vi "Set Reader Timestamp.vi"(9 "timestamp":timestamp format="%<%H:%M:%S%6u\n%x>T", 10 "ID":string="Reader", 11 "data attributes in":variant) -> (3 "data attributes out":variant)   [LabVIEW 2017]
uses:
  <vilib>/Utility/error.llb/whitespace.ctl
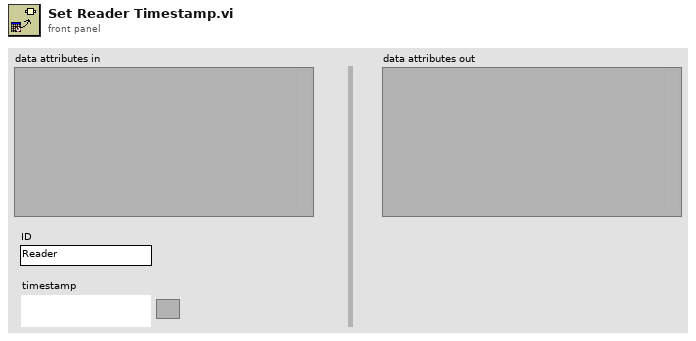
[diagram p1: front panel]
types:
  T1 = typedef "whitespace.ctl" = u16
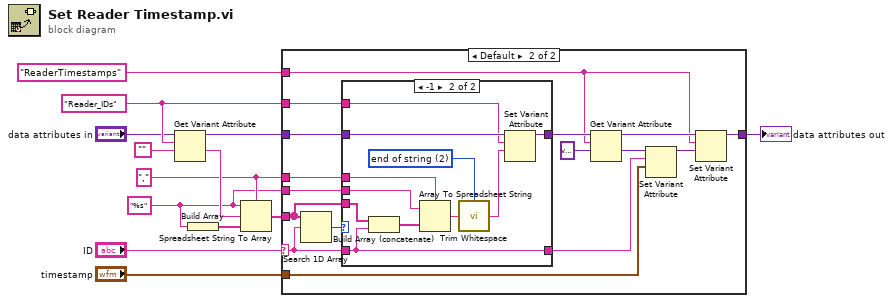
[diagram p0: block diagram]
diagram:
  w7 = "," ("delimiter (Tab)")
  w6 = "Reader_IDs" ("name")
  w5 = "%s" ("format string")
  n1 = Get Variant Attribute(Variant="data attributes in", name=w6, default value (empty Variant)="" ("name")) -> (duplicate Variant=w8:variant, value=w12:string)  [unwired: 1 in, 2 out]
  n2 = Build Array(w5) -> (w11:string[])
  n3 = Spreadsheet String To Array(delimiter (Tab)=w7, format string=w5, spreadsheet string=w12, array type (2D Dbl)=w11) -> (array=w10:string[])
  n4 = case shown="Default" "ID" {
    selector: "ID" -> [_ w27]
    tunnel: w10 -> [_ w28]
    tunnel: [w14 w18] -> w2
    tunnel: w8 -> [w14 w29]
    tunnel: w7 -> [_ w26]
    tunnel: w5 -> [_ w25]
    tunnel: w6 -> [_ w24]
    tunnel: "ReaderTimestamps" ("name") -> [_ w17]
    tunnel: "timestamp" -> [_ w15]
    frame "" {
      # "empty reader ID is used for a ghost reader:\nID \"\" not registered in Reader_IDs\ntimestamp not added to ReaderTimestamps and thus, no hold on data when Delete Stale Samples VI is called"
    }
    frame Default {
      n5 = Search 1D Array(1D array=w28, element=w27) -> (index of element=w30:i32)  [unwired: 1 in]
      n6 = case shown="-1" w30 {
        tunnel: [w32 w43] -> w19
        tunnel: w29 -> [w32 w42]
        tunnel: w28 -> [_ w41]
        tunnel: w27 -> [w31 w35]
        tunnel: w26 -> [_ w39]
        tunnel: w25 -> [_ w38]
        tunnel: w24 -> [_ w37]
        tunnel: [w31 w35] -> w16
        frame Default {
        }
        frame -1 {
          w33 = T1 2 items=["both", "start of string", "end of string"] ("location (both)")
          n7 = Build Array (concatenate)(w41, w35) -> (w40:string[])
          n8 = Array To Spreadsheet String(delimiter (Tab)=w39, array=w40, 3:w38) -> (spreadsheet string=w36:string)
          n9 = call <vilib>:"Trim Whitespace.vi"("string"=w36, "location (both)"=w33) -> ("trimmed string"=w34:string)
          n10 = Set Variant Attribute(Variant=w42, name=w37, value=w34) -> (Variant out=w43:variant)  [unwired: 1 in, 2 out]
        }
      }
      n11 = Get Variant Attribute(Variant=w19, name=w17, default value (empty Variant)=variant ("ReaderTimestamps")) -> (duplicate Variant=w22:variant, value=w23:variant)  [unwired: 1 in, 2 out]
      n12 = Set Variant Attribute(Variant=w23, name=w16, value=w15) -> (Variant out=w21:variant)  [unwired: 1 in, 2 out]
      n13 = Set Variant Attribute(Variant=w22, name=w17, value=w21) -> (Variant out=w18:variant)  [unwired: 1 in, 2 out]
    }
  }
  "data attributes out" <- w2
